vi "minicryo_T-full_202102.vi"() -> (2 "VTI [K]":dbl=9.31008, 3 "Spl [K]":dbl=9.65942)   [LabVIEW 2013]
uses:
  subVI/Global 2.vi
  <vilib>/Analysis/NI_AALPro.lvlib
panel:
  out "Stable?":bool
  in  "stop":bool
  out "Running Sequence":bool
  out "VTI Rate":dbl=0.4518428461335736 format="%#.3g"
  out "Rate":dbl=0.5303975832404774 format="%#.3g"
  in  "Rate":dbl=0.5
  in  "Reset Graph":bool
  in  "Ramp":bool
  in  "Go To":bool
  in  "Set Temp":dbl=10.0
  out "Range":dbl=3.0
  out "VTI":dbl(slide)=46.9 scale=0.0..100.0
  out "T":cluster{"X":dbl[], "Y":dbl[]}[](graph)=[{"X"=[4204.030898399999, 4204.231027299999, 4204.4309592, 4204.632384, 4204.8329014, 4205.0332505999995, 4205.233866099999, 4205.4348291, 4205.6347309, 4205.8353951, 4206.037418299999, 4206.2378935, 4206.4380052999995, 4206.6376684, 4206.838196799999, 4207.0390338, 4207.238357, 4207.4389358, 4207.6389244, 4207.8389028, 4208.0388213999995, 4208.2388605999995, 4208.4383496, 4208.6392350999995, 4208.8409395, 4209.0417325, 4209.2422455999995, 4209.4421716, 4209.6418826, 4209.842302, 4210.0420656999995, 4210.2432989, 4210.442406, 4210.6426186, 4210.8428214, 4211.0434994, 4211.2442437, 4211.443892, 4211.6440931, 4211.8440865, 4212.045375, 4212.2454077, 4212.445538999999, 4212.6465524, 4212.8465418, 4213.046558, 4213.2465348999995, 4213.4464892, 4213.6463585, 4213.8464248, 4214.0479083, 4214.2489233999995, 4214.4484176999995, 4214.649525299999, 4214.851183, 4215.0509592, 4215.2507964999995, 4215.450776, 4215.6509992, 4215.8508409, 4216.050977299999, 4216.2509423, 4216.4514733, 4216.6529347, 4216.854168899999, 4217.0550366, 4217.2544086, 4217.4553365, 4217.6560443, 4217.8560535999995, 4218.0558605, 4218.2560809999995, 4218.4553027, 4218.657004799999, 4218.8579349, 4219.0582892, 4219.257868, 4219.4574629, 4219.6573557], "Y"=[9.18214, 9.18449, 9.18685, 9.18916, 9.19144, 9.1937, 9.19598, 9.19809, 9.2001, 9.20239, 9.20465, 9.20678, 9.20882, 9.21085, 9.21272, 9.21463, 9.21645, 9.21831, 9.22005, 9.22177, 9.22347, 9.22515, 9.22671, 9.22826, 9.22981, 9.23127, 9.23259, 9.2339, 9.23515, 9.23639, 9.23767, 9.23909, 9.24053, 9.24185, 9.2431, 9.24439, 9.24556, 9.24682, 9.24801, 9.24932, 9.25062, 9.25202, 9.25345, 9.25482, 9.25621, 9.25767, 9.25918, 9.26068, 9.26217, 9.26374, 9.26529, 9.26685, 9.26846, 9.2701, 9.27169, 9.27328, 9.27486, 9.27645, 9.27803, 9.27964, 9.2812, 9.28274, 9.28433, 9.28609, 9.28773, 9.28938, 9.29107, 9.29271, 9.29438, 9.29605, 9.29774, 9.2994, 9.30097, 9.30247, 9.30394, 9.30545, 9.30691, 9.30844, 9.31008]}, {"X"=[4204.030898399999, 4204.231027299999, 4204.4309592, 4204.632384, 4204.8329014, 4205.0332505999995, 4205.233866099999, 4205.4348291, 4205.6347309, 4205.8353951, 4206.037418299999, 4206.2378935, 4206.4380052999995, 4206.6376684, 4206.838196799999, 4207.0390338, 4207.238357, 4207.4389358, 4207.6389244, 4207.8389028, 4208.0388213999995, 4208.2388605999995, 4208.4383496, 4208.6392350999995, 4208.8409395, 4209.0417325, 4209.2422455999995, 4209.4421716, 4209.6418826, 4209.842302, 4210.0420656999995, 4210.2432989, 4210.442406, 4210.6426186, 4210.8428214, 4211.0434994, 4211.2442437, 4211.443892, 4211.6440931, 4211.8440865, 4212.045375, 4212.2454077, 4212.445538999999, 4212.6465524, 4212.8465418, 4213.046558, 4213.2465348999995, 4213.4464892, 4213.6463585, 4213.8464248, 4214.0479083, 4214.2489233999995, 4214.4484176999995, 4214.649525299999, 4214.851183, 4215.0509592, 4215.2507964999995, 4215.450776, 4215.6509992, 4215.8508409, 4216.050977299999, 4216.2509423, 4216.4514733, 4216.6529347, 4216.854168899999, 4217.0550366, 4217.2544086, 4217.4553365, 4217.6560443, 4217.8560535999995, 4218.0558605, 4218.2560809999995, 4218.4553027, 4218.657004799999, 4218.8579349, 4219.0582892, 4219.257868, 4219.4574629, 4219.6573557], "Y"=[9.50261, 9.50508, 9.50755, 9.5095, 9.51232, 9.51564, 9.5181, 9.52127, 9.52353, 9.52773, 9.52985, 9.53237, 9.53378, 9.53555, 9.53901, 9.54188, 9.54449, 9.54641, 9.54792, 9.54933, 9.55335, 9.55549, 9.55871, 9.56214, 9.56318, 9.56586, 9.56687, 9.56873, 9.57072, 9.57162, 9.57379, 9.57687, 9.58018, 9.5823, 9.58495, 9.58667, 9.58745, 9.58839, 9.58911, 9.59111, 9.59322, 9.59607, 9.59767, 9.59894, 9.6008, 9.60204, 9.60328, 9.605, 9.60693, 9.60817, 9.60977, 9.61135, 9.6134, 9.61627, 9.61854, 9.62061, 9.62163, 9.62284, 9.62393, 9.62645, 9.62846, 9.62946, 9.63039, 9.63239, 9.63515, 9.63699, 9.63858, 9.63994, 9.642, 9.64486, 9.64862, 9.65129, 9.65236, 9.65324, 9.65559, 9.65607, 9.65744, 9.65857, 9.65942]}] caption="XY Graph"
  out "Set VTI [K]":dbl=9.645
  # "Heaters"
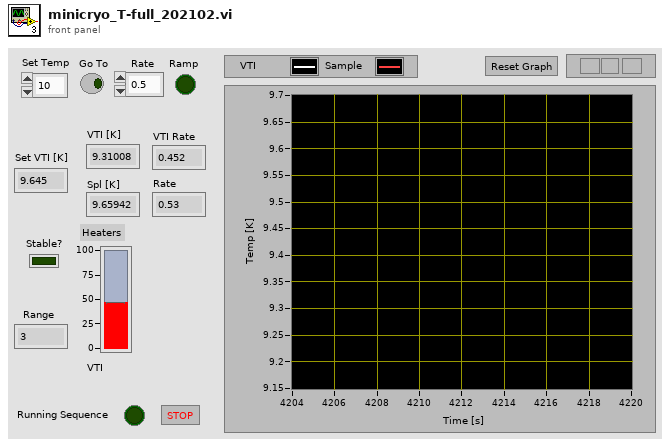
[diagram p1: front panel]
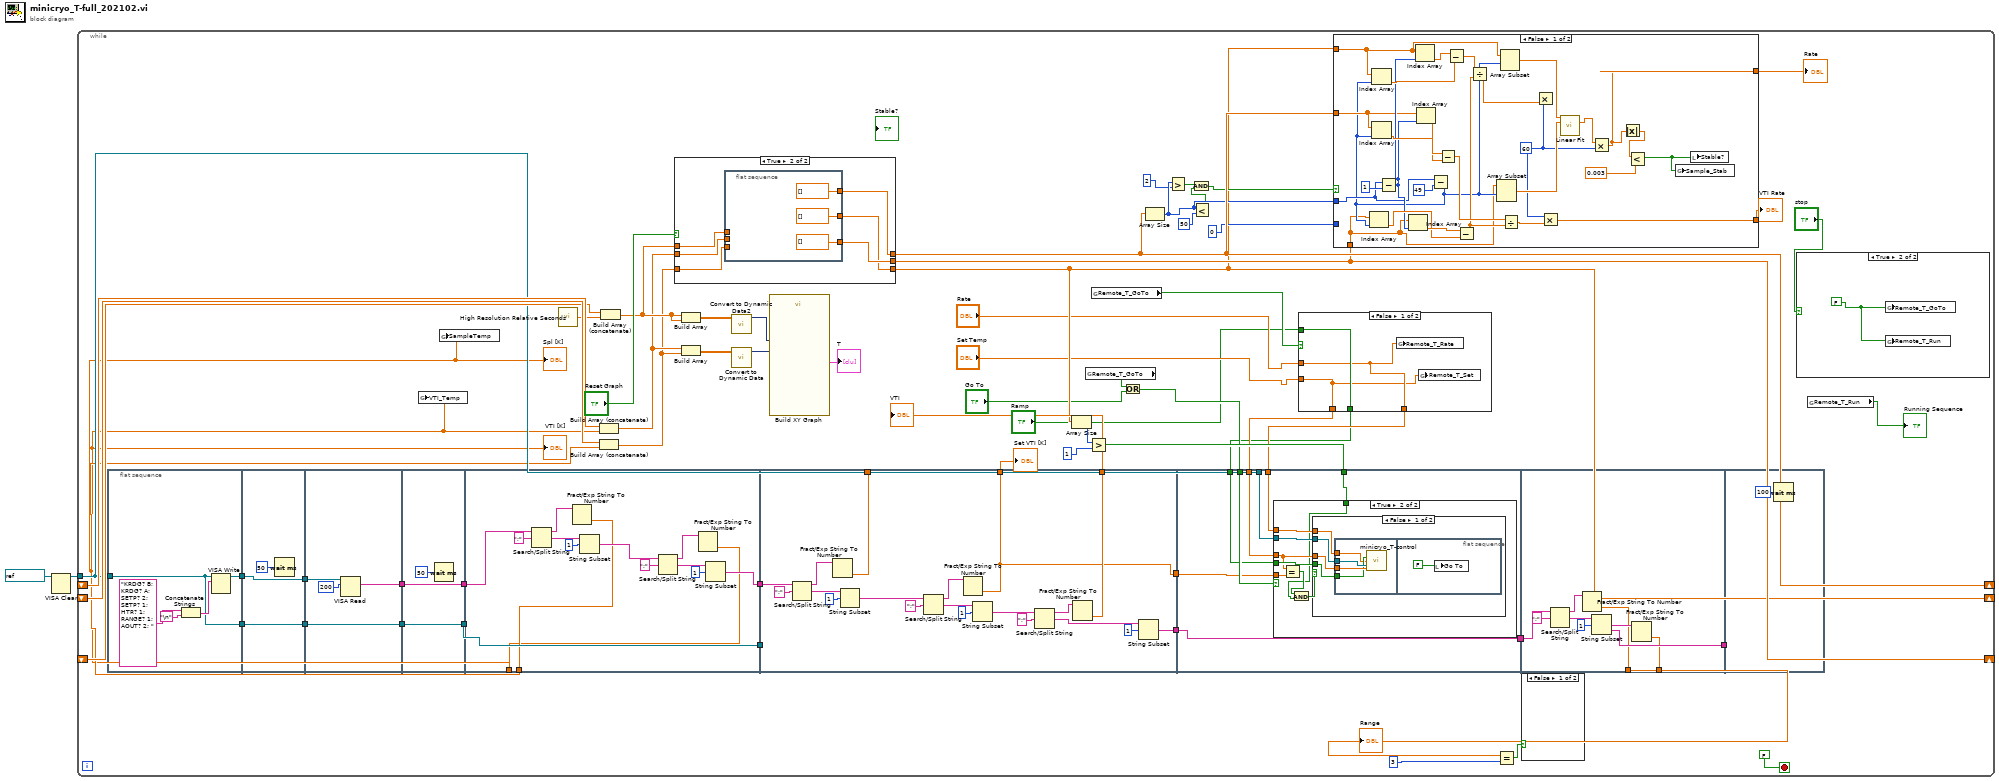
[diagram p0: block diagram]
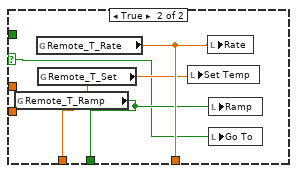
[diagram p3: hidden frame]
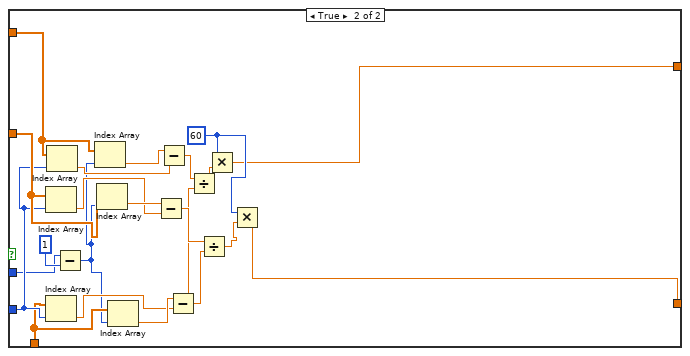
[diagram p4: hidden frame]
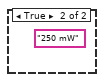
[diagram p6: hidden frame]
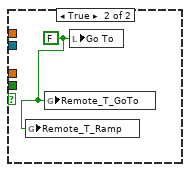
[diagram p8: hidden frame]
diagram:
  n1 = VISA Clear(VISA resource name=refnum<visa-resource-name> "COM5" ("Lakeshore Address")) -> (VISA resource name out=w2:refnum<visa-resource-name>)  [unwired: 1 in, 1 out]
  n2 = while {
    tunnel: w2 -> [w33]
    shift-right: [w19] -> _
    shift-left: _ -> [w61]
    shift-right: [w31] -> _
    shift-left: _ -> [w60]
    shift-right: [w28] -> _
    shift-left: _ -> [w58]
    stop <- FALSE stop-if-true
    n3 = flat-sequence {
      tunnel: w33 -> [w136]
      tunnel: [w136] -> w43
      tunnel: [w135] -> w40
      tunnel: w43 -> [w142]
      tunnel: [w142] -> w42
      tunnel: [w140] -> w41
      tunnel: w40 -> [w140]
      tunnel: [w146] -> w49
      tunnel: w42 -> [w146]
      tunnel: w41 -> [w144]
      tunnel: [w143] -> w37
      tunnel: [w149] -> w65
      tunnel: w49 -> [w149]
      tunnel: [w147] -> w38
      tunnel: w37 -> [w147]
      tunnel: w65 -> [w163]
      tunnel: [w150] -> w15
      tunnel: [w151] -> w16
      tunnel: [w163] -> w62
      tunnel: [w152] -> w39
      tunnel: w38 -> [w154]
      tunnel: [w182] -> w35
      tunnel: [w164] -> w32
      tunnel: [w180] -> w52
      tunnel: [w164] -> w64
      tunnel: [w181] -> _
      tunnel: w39 -> [w166]
      tunnel: w62 -> [_]
      tunnel: w35 -> [w190]
      tunnel: [w190] -> w34
      tunnel: w12 -> [w189]
      tunnel: w33 -> [w188]
      tunnel: w7 -> [w187]
      tunnel: w5 -> [w186]
      tunnel: w9 -> [w185]
      tunnel: w32 -> [w184]
      tunnel: w17 -> [w183]
      tunnel: [w216] -> w36
      tunnel: [w215] -> _
      tunnel: w34 -> [w209]
      tunnel: [w214] -> w44
      tunnel: w36 -> [_]
      frame #0 {
        n4 = Concatenate Strings("KRDG? B; KRDG? A; SETP? 2; SETP? 1; HTR? 1; RANGE? 1; AOUT? 2; " ("write buffer"), "\n") -> (w137:string)
        n5 = VISA Write(VISA resource name=w136, write buffer=w137) -> (VISA resource name out=w135:refnum<visa-resource-name>)  [unwired: 1 in, 2 out]
      }
      frame #1 {
        n6 = Wait (ms)(milliseconds to wait=50) -> ()  [unwired: 1 out]
      }
      frame #2 {
        n7 = VISA Read(VISA resource name=w144, byte count=u32 200) -> (read buffer=w143:string)  [unwired: 1 in, 3 out]
      }
      frame #3 {
        n8 = Wait (ms)(milliseconds to wait=50) -> ()  [unwired: 1 out]
      }
      frame #4 {
        n9 = Search/Split String(string=w154, search string/char (-)=";") -> (substring before match=w159:string, match + rest of string=w161:string)  [unwired: 1 in, 1 out]
        n10 = Fract/Exp String To Number(string=w159) -> (number=w151:dbl)  [unwired: 3 in, 1 out]
        n11 = String Subset(string=w161, offset (0)=u32 1 ("byte count")) -> (substring=w153:string)  [unwired: 1 in]
        n12 = Search/Split String(string=w153, search string/char (-)=";") -> (substring before match=w155:string, match + rest of string=w157:string)  [unwired: 1 in, 1 out]
        n13 = Fract/Exp String To Number(string=w155) -> (number=w150:dbl)  [unwired: 3 in, 1 out]
        n14 = String Subset(string=w157, offset (0)=u32 1 ("byte count")) -> (substring=w152:string)  [unwired: 1 in]
      }
      frame #5 {
        n15 = Search/Split String(string=w166, search string/char (-)=";") -> (substring before match=w165:string, match + rest of string=w168:string)  [unwired: 1 in, 1 out]
        n16 = Fract/Exp String To Number(string=w165) -> (number=w181:dbl)  [unwired: 3 in, 1 out]
        n17 = String Subset(string=w168, offset (0)=u32 1 ("byte count")) -> (substring=w171:string)  [unwired: 1 in]
        n18 = Search/Split String(string=w171, search string/char (-)=";") -> (substring before match=w170:string, match + rest of string=w173:string)  [unwired: 1 in, 1 out]
        n19 = Fract/Exp String To Number(string=w170) -> (number=w164:dbl)  [unwired: 3 in, 1 out]
        n20 = String Subset(string=w173, offset (0)=u32 1 ("byte count")) -> (substring=w176:string)  [unwired: 1 in]
        n21 = Search/Split String(string=w176, search string/char (-)=";") -> (substring before match=w175:string, match + rest of string=w178:string)  [unwired: 1 in, 1 out]
        n22 = Fract/Exp String To Number(string=w175) -> (number=w180:dbl)  [unwired: 3 in, 1 out]
        n23 = String Subset(string=w178, offset (0)=u32 1 ("byte count")) -> (substring=w182:string)  [unwired: 1 in]
      }
      frame #6 {
        n24 = case shown="True" w189 {
          tunnel: w188 -> [_ w198]
          tunnel: w187 -> [_ w194]
          tunnel: w186 -> [_ w197]
          tunnel: w185 -> [_ w196]
          tunnel: w184 -> [_ w195]
          tunnel: w183 -> [_ w192]
          frame False {
          }
          frame True {
            n25 = Equal?(x=w194, y=w195) -> (x = y?=w193:bool)
            n26 = And(x=w193, y=w192) -> (x .and. y?=w191:bool)
            n27 = case shown="False" w191 {
              tunnel: w198 -> [w202 _]
              tunnel: w194 -> [w201 _]
              tunnel: w197 -> [w200 _]
              tunnel: w196 -> [w199 _]
              frame False {
                n28 = flat-sequence {
                  tunnel: w202 -> [w206]
                  tunnel: w201 -> [w205]
                  tunnel: w200 -> [w204]
                  tunnel: w199 -> [w203]
                  frame #0 {
                    n29 = call "minicryo_T-control.vi"("Ramp Mode"=w204, "Rate  [K/min]"=w203, "VISA resource name out"=w206, "Set Sample Temp [K]"=w205) -> ()  [unwired: 12 in]
                  }
                  frame #1 {
                    n30 = local write "Go To"(FALSE) -> ()
                  }
                }
              }
              frame True {
                w208 = FALSE
                n31 = global write "Global 2.vi" "Remote_T_Ramp"(w208) -> ()
                n32 = global write "Global 2.vi" "Remote_T_GoTo"(w208) -> ()
                n33 = local write "Go To"(w208) -> ()
              }
            }
          }
        }
      }
      frame #7 {
        n34 = Search/Split String(string=w209, search string/char (-)=";") -> (substring before match=w210:string, match + rest of string=w212:string)  [unwired: 1 in, 1 out]
        n35 = Fract/Exp String To Number(string=w210) -> (number=w214:dbl)  [unwired: 3 in, 1 out]
        n36 = String Subset(string=w212, offset (0)=u32 1 ("byte count")) -> (substring=w216:string)  [unwired: 1 in]
        n37 = Fract/Exp String To Number(string=w216) -> (number=w215:dbl)  [unwired: 3 in, 1 out]
      }
      frame #8 {
        n38 = Wait (ms)(milliseconds to wait=100) -> ()  [unwired: 1 out]
      }
    }
    n39 = global write "Global 2.vi" "VTI_Temp"(w15) -> ()
    n40 = global write "Global 2.vi" "SampleTemp"(w16) -> ()
    n41 = call <vilib>:"High Resolution Relative Seconds.vi"() -> ("relative seconds"=w57:dbl)
    n42 = Build Array (concatenate)(w60, w15) -> (w46:dbl[])
    n43 = Build Array (concatenate)(w61, w16) -> (w45:dbl[])
    n44 = Build Array (concatenate)(w58, w57) -> (w47:dbl[])
    n45 = case shown="True" "Reset Graph" {
      tunnel: w47 -> [w125 w131]
      tunnel: [w125 w130] -> w28
      tunnel: w46 -> [w124 w129]
      tunnel: [w124 w128] -> w31
      tunnel: w45 -> [w123 w127]
      tunnel: [w123 w126] -> w19
      frame False {
      }
      frame True {
        n46 = flat-sequence {
          tunnel: w131 -> [_]
          tunnel: w129 -> [_]
          tunnel: w127 -> [_]
          tunnel: [dbl[] []] -> w128
          tunnel: [dbl[] []] -> w130
          tunnel: [dbl[] []] -> w126
          frame #0 {
          }
        }
      }
    }
    n47 = Build Array(w47, w47) -> (w54:dbl[][])
    n48 = Build Array(w46, w45) -> (w56:dbl[][])
    n49 = call "Convert to Dynamic Data2"("2D Array"=w54) -> ("Dynamic Data Type"=w53:dynamicdata)  [unwired: 3 in]
    n50 = call "Convert to Dynamic Data"("2D Array"=w56) -> ("Dynamic Data Type"=w55:dynamicdata)  [unwired: 3 in]
    n51 = call "Build XY Graph"("Y Input"=w55, "X Input"=w53) -> ("XY Graph"=→"T":cluster{"X":dbl[], "Y":dbl[]}[])  [unwired: 8 in, 1 out]
    n52 = Array Size(array=w19) -> (size(s)=w20:i32)
    n53 = global read "Global 2.vi" "Remote_T_GoTo"() -> (w14:bool)
    n54 = Greater?(x=w20, y=1) -> (0:w17:bool)
    n55 = global read "Global 2.vi" "Remote_T_GoTo"() -> (w11:bool)
    n56 = Or(x=w14, y="Go To") -> (x .or. y?=w12:bool)
    n57 = Array Size(array=w31) -> (size(s)=w25:i32)
    n58 = Greater?(x=w25, y=2) -> (0:w27:bool)
    n59 = Less?(x=w25, y=50) -> (x < y?=w23:bool)
    n60 = And(x=w27, y=w23) -> (x .and. y?=w26:bool)
    n61 = case shown="False" w11 {
      selector: w11 -> [_ w70]
      tunnel: "Rate" -> [w68 _]
      tunnel: [w68 w73] -> w9
      tunnel: "Set Temp" -> [w67 _]
      tunnel: [w67 w72] -> w7
      tunnel: "Ramp" -> [w69 _]
      tunnel: [w69 w71] -> w5
      frame False {
        n62 = global write "Global 2.vi" "Remote_T_Rate"(w68) -> ()
        n63 = global write "Global 2.vi" "Remote_T_Set"(w67) -> ()
      }
      frame True {
        n64 = global read "Global 2.vi" "Remote_T_Ramp"() -> (w71:bool)
        n65 = global read "Global 2.vi" "Remote_T_Rate"() -> (w73:dbl)
        n66 = global read "Global 2.vi" "Remote_T_Set"() -> (w72:dbl)
        n67 = local write "Set Temp"(w72) -> ()
        n68 = local write "Rate"(w73) -> ()
        n69 = local write "Ramp"(w71) -> ()
        n70 = local write "Go To"(w70) -> ()
      }
    }
    n71 = case shown="False" w26 {
      tunnel: w31 -> [w85 w122]
      tunnel: 0 -> [_ w121]
      tunnel: w25 -> [w87 w105]
      tunnel: w28 -> [w82 w119]
      tunnel: w19 -> [w84 w120]
      tunnel: [w76 w103] -> w22
      tunnel: [w88 w102] -> w21
      frame False {
        w79 = 60
        n72 = Subtract(x=w87, y=1) -> (x-y=w89:i32)
        n73 = Index Array(array=w82, index=w89) -> (element=w101:dbl)
        n74 = Index Array(array=w84, index=w89) -> (element=w97:dbl)
        n75 = Index Array(array=w85, index=w89) -> (element=w99:dbl)
        n76 = Subtract(x=w87, y=49) -> (x-y=w83:i32)
        n77 = Index Array(array=w82, index=w83) -> (element=w100:dbl)
        n78 = Index Array(array=w84, index=w83) -> (element=w96:dbl)
        n79 = Index Array(array=w85, index=w83) -> (element=w98:dbl)
        n80 = Subtract(x=w99, y=w98) -> (x-y=w94:dbl)
        n81 = Subtract(x=w97, y=w96) -> (x-y=w95:dbl)
        n82 = Subtract(x=w101, y=w100) -> (x-y=w93:dbl)
        n83 = Divide(x=w95, y=w93) -> (x/y=w92:dbl)
        n84 = Array Subset(array=w82, index=w83) -> (w80:dbl[])  [unwired: 1 in]
        n85 = Array Subset(array=w84, index=w83) -> (w81:dbl[])  [unwired: 1 in]
        n86 = Divide(x=w94, y=w93) -> (x/y=w91:dbl)
        n87 = Multiply(x=w79, y=w92) -> ()  [unwired: 1 out]
        n88 = Multiply(x=w79, y=w91) -> (x*y=w88:dbl)
        n89 = call <vilib>:"Linear Fit.vi"("Y"=w81, "X"=w80) -> ("slope"=w78:dbl)  [unwired: 9 in, 4 out]
        n90 = Multiply(x=w78, y=w79) -> (x*y=w76:dbl)
        n91 = Absolute Value(x=w76) -> (abs(x)=w75:dbl)
        n92 = Less?(x=w75, y=0.003) -> (x < y?=w74:bool)
        n93 = global write "Global 2.vi" "Sample_Stab"(w74) -> ()
        n94 = local write "Stable?"(w74) -> ()
      }
      frame True {
        w108 = 60
        n95 = Index Array(array=w122, index=w121) -> (element=w115:dbl)
        n96 = Index Array(array=w119, index=w121) -> (element=w117:dbl)
        n97 = Index Array(array=w120, index=w121) -> (element=w113:dbl)
        n98 = Subtract(x=w105, y=1) -> (x-y=w104:i32)
        n99 = Index Array(array=w120, index=w104) -> (element=w114:dbl)
        n100 = Index Array(array=w122, index=w104) -> (element=w116:dbl)
        n101 = Index Array(array=w119, index=w104) -> (element=w118:dbl)
        n102 = Subtract(x=w116, y=w115) -> (x-y=w111:dbl)
        n103 = Subtract(x=w114, y=w113) -> (x-y=w112:dbl)
        n104 = Subtract(x=w118, y=w117) -> (x-y=w110:dbl)
        n105 = Divide(x=w112, y=w110) -> (x/y=w109:dbl)
        n106 = Divide(x=w111, y=w110) -> (x/y=w107:dbl)
        n107 = Multiply(x=w108, y=w109) -> (x*y=w103:dbl)
        n108 = Multiply(x=w108, y=w107) -> (x*y=w102:dbl)
      }
    }
    "Rate" <- w22
    "VTI Rate" <- w21
    n109 = Equal?(x=w44, y=3) -> (x = y?=w50:bool)
    n110 = case shown="False" w50 {
      frame False {
      }
      frame True {
        (unwired) "250 mW"
      }
    }
    n111 = case shown="True" "stop" {
      frame False {
      }
      frame True {
        w66 = FALSE
        n112 = global write "Global 2.vi" "Remote_T_GoTo"(w66) -> ()
        n113 = global write "Global 2.vi" "Remote_T_Run"(w66) -> ()
      }
    }
    n114 = global read "Global 2.vi" "Remote_T_Run"() -> (→"Running Sequence":bool)
    "Spl [K]" <- w16
    "VTI [K]" <- w15
    "Set VTI [K]" <- w64
    "VTI" <- w52
    "Range" <- w44
  }
